vi "Read Text.vi"(9 "String in":refnum<class "String.lvclass">) -> (3 "String out":refnum<class "String.lvclass">, 4 "Text":refnum<class "Text.lvclass">)   [LabVIEW 2014, in "String.lvclass"]
uses:
  String.lvclass
  Text/Text.lvclass
  String.lvclass/String.ctl
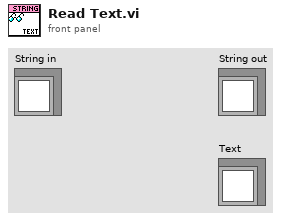
[diagram p1: front panel]
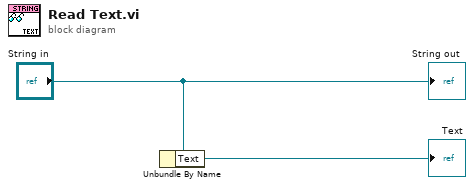
[diagram p0: block diagram]
diagram:
  n1 = Unbundle By Name("String in") -> ("Text"=→"Text":refnum<class "Text.lvclass">)
  "String out" <- "String in"
